vi "niRFUtil MT UTIL Validate Pack Bits.vi"(0 "bits per integer":i32=1, 5 "input bit stream":i8[](array[numeric]), 7 "integer format":enum16{"Unsigned", "Signed"}(ring)) -> (15 "error out":errorcluster)   [LabVIEW 2015, in "niRFUtil.lvlib"]
uses:
  niRFUtil.lvlib
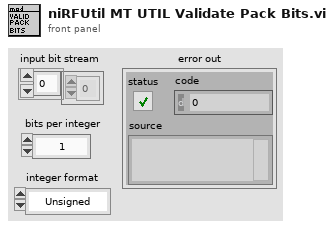
[diagram p1: front panel]
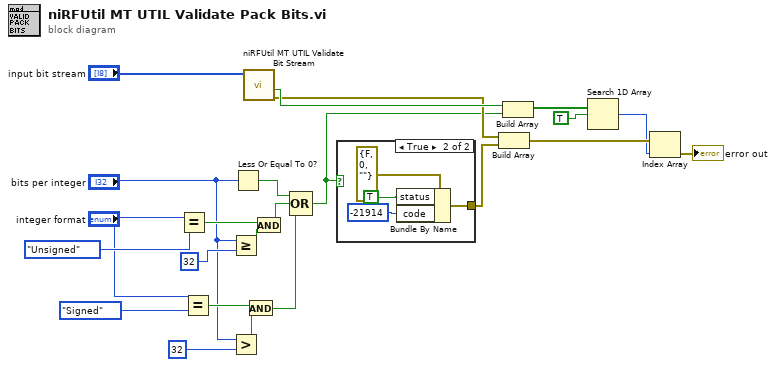
[diagram p0: block diagram]
diagram:
  n1 = Equal?(x="integer format", y=enum16{"Unsigned", "Signed"}."Unsigned") -> (x = y?=w11:bool)
  n2 = Equal?(x="integer format", y=enum16{"Unsigned", "Signed"}."Signed") -> (x = y?=w8:bool)
  n3 = Greater Or Equal?(x="bits per integer", y=32) -> (x >= y?=w10:bool)
  n4 = Greater?(x="bits per integer", y=32) -> (0:w7:bool)
  n5 = Less Or Equal To 0?(x="bits per integer") -> (x <= 0?=w14:bool)
  n6 = call "niRFUtil MT UTIL Validate Bit Stream.vi"("Input Bit Stream"="input bit stream") -> ("error out"=w16:errorcluster, "error?"=w17:bool)  [unwired: 9 in]
  n7 = And(x=w8, y=w7) -> (x .and. y?=w5:bool)
  n8 = And(x=w11, y=w10) -> (x .and. y?=w6:bool)
  n9 = Compound Arithmetic op=OR(w14, w6, w5) -> (w13:bool)
  n10 = case shown="True" w13 {
    tunnel: [_ w24] -> w15
    frame False {
    }
    frame True {
      n11 = Bundle By Name(cluster=errorcluster {"status"=FALSE, "code"=0, "source"=""} ("error out"), "status"=TRUE, "code"=-21914) -> (w24:errorcluster)
    }
  }
  n12 = Build Array(w16, w15) -> (w20:errorcluster[])
  n13 = Build Array(w17, w13) -> (w22:bool[])
  n14 = Search 1D Array(1D array=w22, element=TRUE) -> (index of element=w19:i32)  [unwired: 1 out]
  n15 = Index Array(array=w20, index=w19) -> (element=→"error out":errorcluster)
